vi "ConfigureMeasurement.vi"(4 "Trace":u32=1, 6 "Meas Param":enum16{"S21", "S12", "S11", "S22"}(ring), 7 "Window":u32=1, 8 "error in (no error)":errorcluster, 9 "Meas Name":string="MY_MEAS", 10 "Channel":u32=1, 11 "NetA_AgNA in":refnum<class "NetA_AgNA.lvclass">) -> (0 "error out":errorcluster, 3 "NetA_AgNA out":refnum<class "NetA_AgNA.lvclass">)   [LabVIEW 2014, in "NetA_AgNA.lvclass"]
doc: "Creates a measurement. Alternative to the options in Agilent NA.lvlib."
uses:
  NetA_AgNA.lvclass
  NetA_AgNA.lvclass/NetA_AgNA.ctl
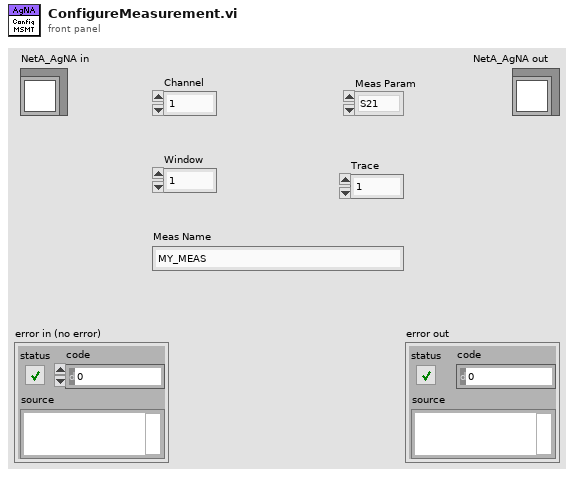
[diagram p1: front panel]
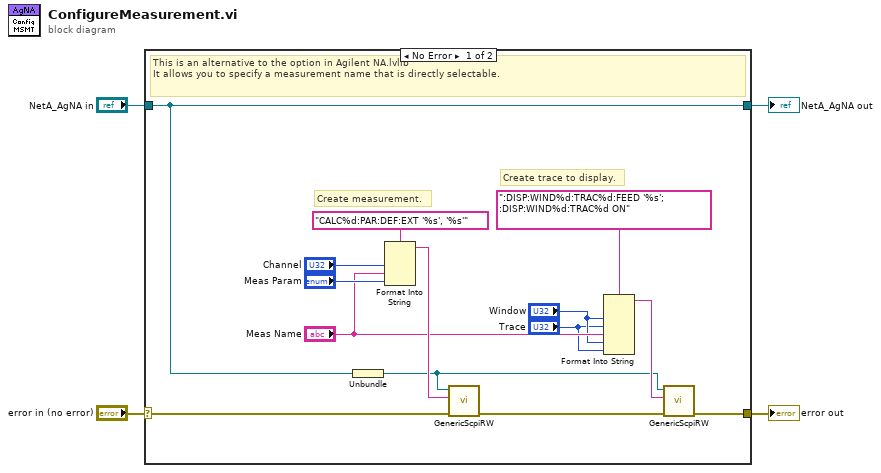
[diagram p0: block diagram]
diagram:
  n1 = case shown="No Error" "error in (no error)" {
    selector: "error in (no error)" -> [w18 w20]
    tunnel: [w16 w20] -> w3
    tunnel: "NetA_AgNA in" -> [w6 w19]
    tunnel: [w6 w19] -> w1
    frame No Error {
      # "Create measurement."
      # "Create trace to display."
      # "This is an alternative to the option in Agilent NA.lvlib\nIt allows you to specify a measurement name that is directly selectable."
      n2 = Unbundle(w6) -> (w5:refnum<k15>)
      n3 = Format Into String(format string="CALC%d:PAR:DEF:EXT '%s', '%s'" ("Get Dir List"), "Channel", "Meas Name", "Meas Param") -> (resulting string=w12:string)  [unwired: 2 in, 1 out]
      n4 = call "GenericScpiRW.vi"("error in (no error)"=w18, "SCPI Command"=w12, "resource name"=w5) -> ("error out"=w17:errorcluster)  [unwired: 7 in, 1 out]
      n5 = Format Into String(format string=":DISP:WIND%d:TRAC%d:FEED '%s'; :DISP:WIND%d:TRAC%d ON" ("Get Dir List"), "Window", "Trace", "Meas Name", "Window", "Trace") -> (resulting string=w7:string)  [unwired: 2 in, 1 out]
      n6 = call "GenericScpiRW.vi"("error in (no error)"=w17, "SCPI Command"=w7, "resource name"=w5) -> ("error out"=w16:errorcluster)  [unwired: 7 in, 1 out]
    }
    frame Error {
    }
  }
  "error out" <- w3
  "NetA_AgNA out" <- w1
